vi "get_settings_cluster.vi"(8 "error in (no error)":errorcluster, 11 "GenericPlugin in":refnum<class "ScanHeadMH100729FPGA.lvclass">) -> (0 "error out":errorcluster, 2 "settings cluster":variant, 3 "GenericPlugin out":refnum<class "ScanHeadMH100729FPGA.lvclass">)   [LabVIEW 2010, in "ScanHeadMH100729FPGA.lvclass"]
uses:
  ScanHeadMH100729FPGA.lvclass
  ScanHeadMH100729FPGA.lvclass/ScanHeadMH100729FPGA.ctl
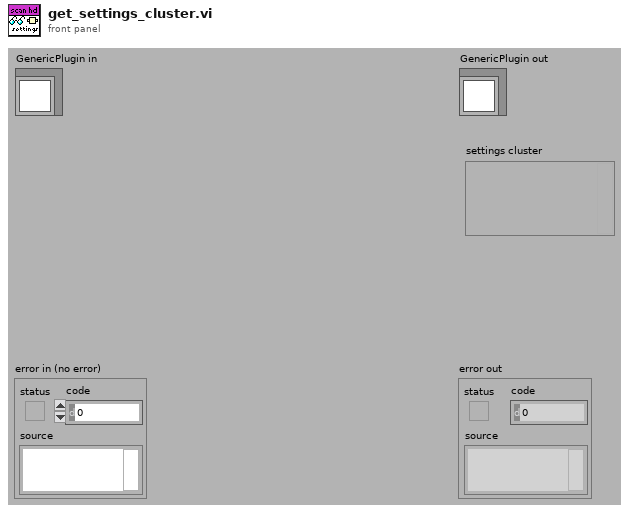
[diagram p1: front panel]
types:
  T1 = typedef "ScanHeadMH100729FPGA.lvclass/settings_cluster.ctl" = cluster{"Zoom":dbl, "Intensity":dbl, "AngleZ":dbl[unit], "AngleX":dbl[unit], "OffsetX":dbl[unit], "OffsetY":dbl[unit], "OffsetZ":dbl[unit], "ScatteringLength":dbl[unit], "intensity adjustment mode":T2, "translation mode":T3}
  T2 = typedef "ScanHeadMH100729FPGA.lvclass/intensity_adjustment_enum.ctl" = enum16{"manual", "look-up", "exponential"}
  T3 = typedef "ScanHeadMH100729FPGA.lvclass/translation_mode_enum.ctl" = enum16{"scan signal offset", "stage"}
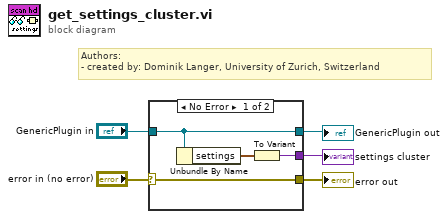
[diagram p0: block diagram]
diagram:
  # "Authors: \n- created by: Dominik Langer, University of Zurich, Switzerland"
  n1 = case shown="No Error" "error in (no error)" {
    selector: "error in (no error)" -> [w7 w10]
    tunnel: "GenericPlugin in" -> [w6 w11]
    tunnel: [w8 _] -> w3
    tunnel: [w7 w10] -> w2
    tunnel: [w6 w11] -> w1
    frame No Error {
      n2 = Unbundle By Name(w6) -> ("settings"=w9:T1)
      n3 = To Variant(anything=w9) -> (Variant=w8:variant)
    }
    frame Error {
    }
  }
  "error out" <- w2
  "GenericPlugin out" <- w1
  "settings cluster" <- w3
